vi "XML_Data.vi"(8 "Data Input Array":dbl[](array[numeric]), 9 "Data Tag Names Array":string[](array[string])=["DATA_1", "DATA_2", "DATA_3", "DATA_4"], 10 "XML File Path":path, 11 "DOM document in":refnum<k20>) -> (2 "XML Output":string, 3 "DOM document out":refnum<k20>)   [LabVIEW 2009]
doc: "Parses and Inserts a 1-D array of data into an XML file specified by the file path. The input XML file must have a DATA_SET node. Also, takes a 1-D array of strings to determine the node names for the data tags. The XML_Data VI can take 1-D arrays with 1-6 elements for both the numaric and string arrays, but can be modified to add up to 9 total. \n\nNOTE: If the string and numaric arrays are of different lengths the length of the numaric array will be used to determine the number of data nodes the XML file will have and data node names will be filled in with default values if needed."
uses:
  Program Files/National Instruments/LabVIEW 2009/resource/objmgr/DOMUserDefRef.rc
  <vilib>/xml/NI_XML.lvlib
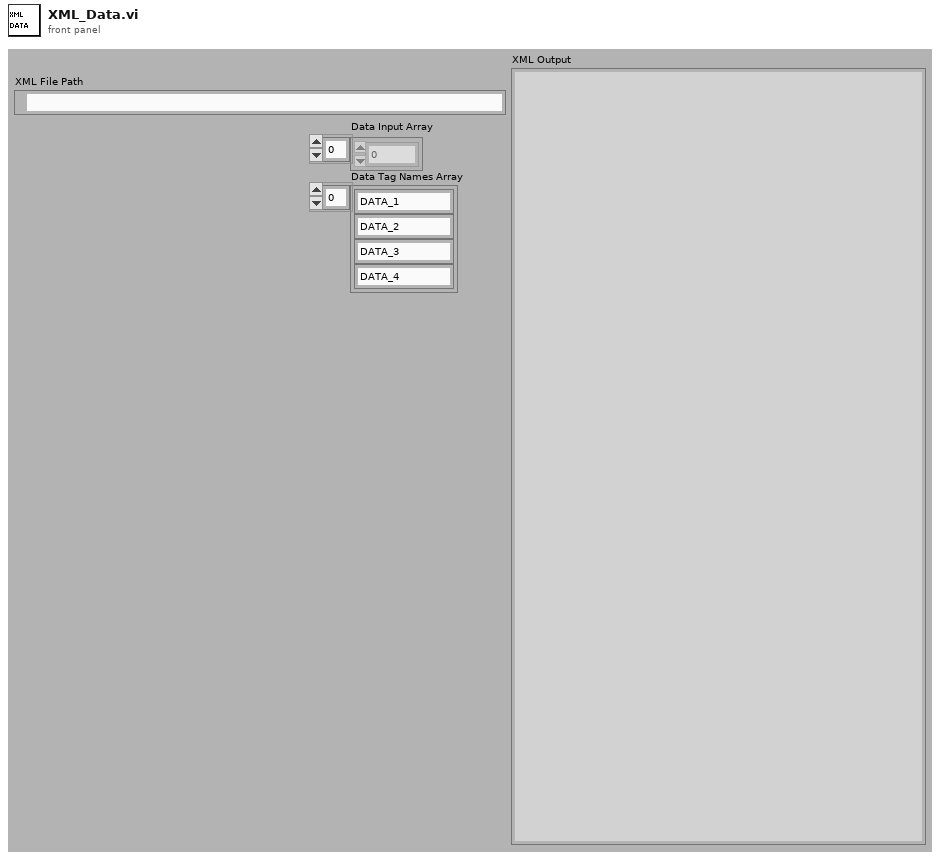
[diagram p1: front panel]
types:
  T1 = cluster{"Data Tag Names Array[0]":string, "Data Tag Names Array[1]":string, "Data Tag Names Array[2]":string, "Data Tag Names Array[3]":string, "Data Tag Names Array[4]":string, "Data Tag Names Array[5]":string, "Data Tag Names Array[6]":string, "Data Tag Names Array[7]":string, "Data Tag Names Array[8]":string}
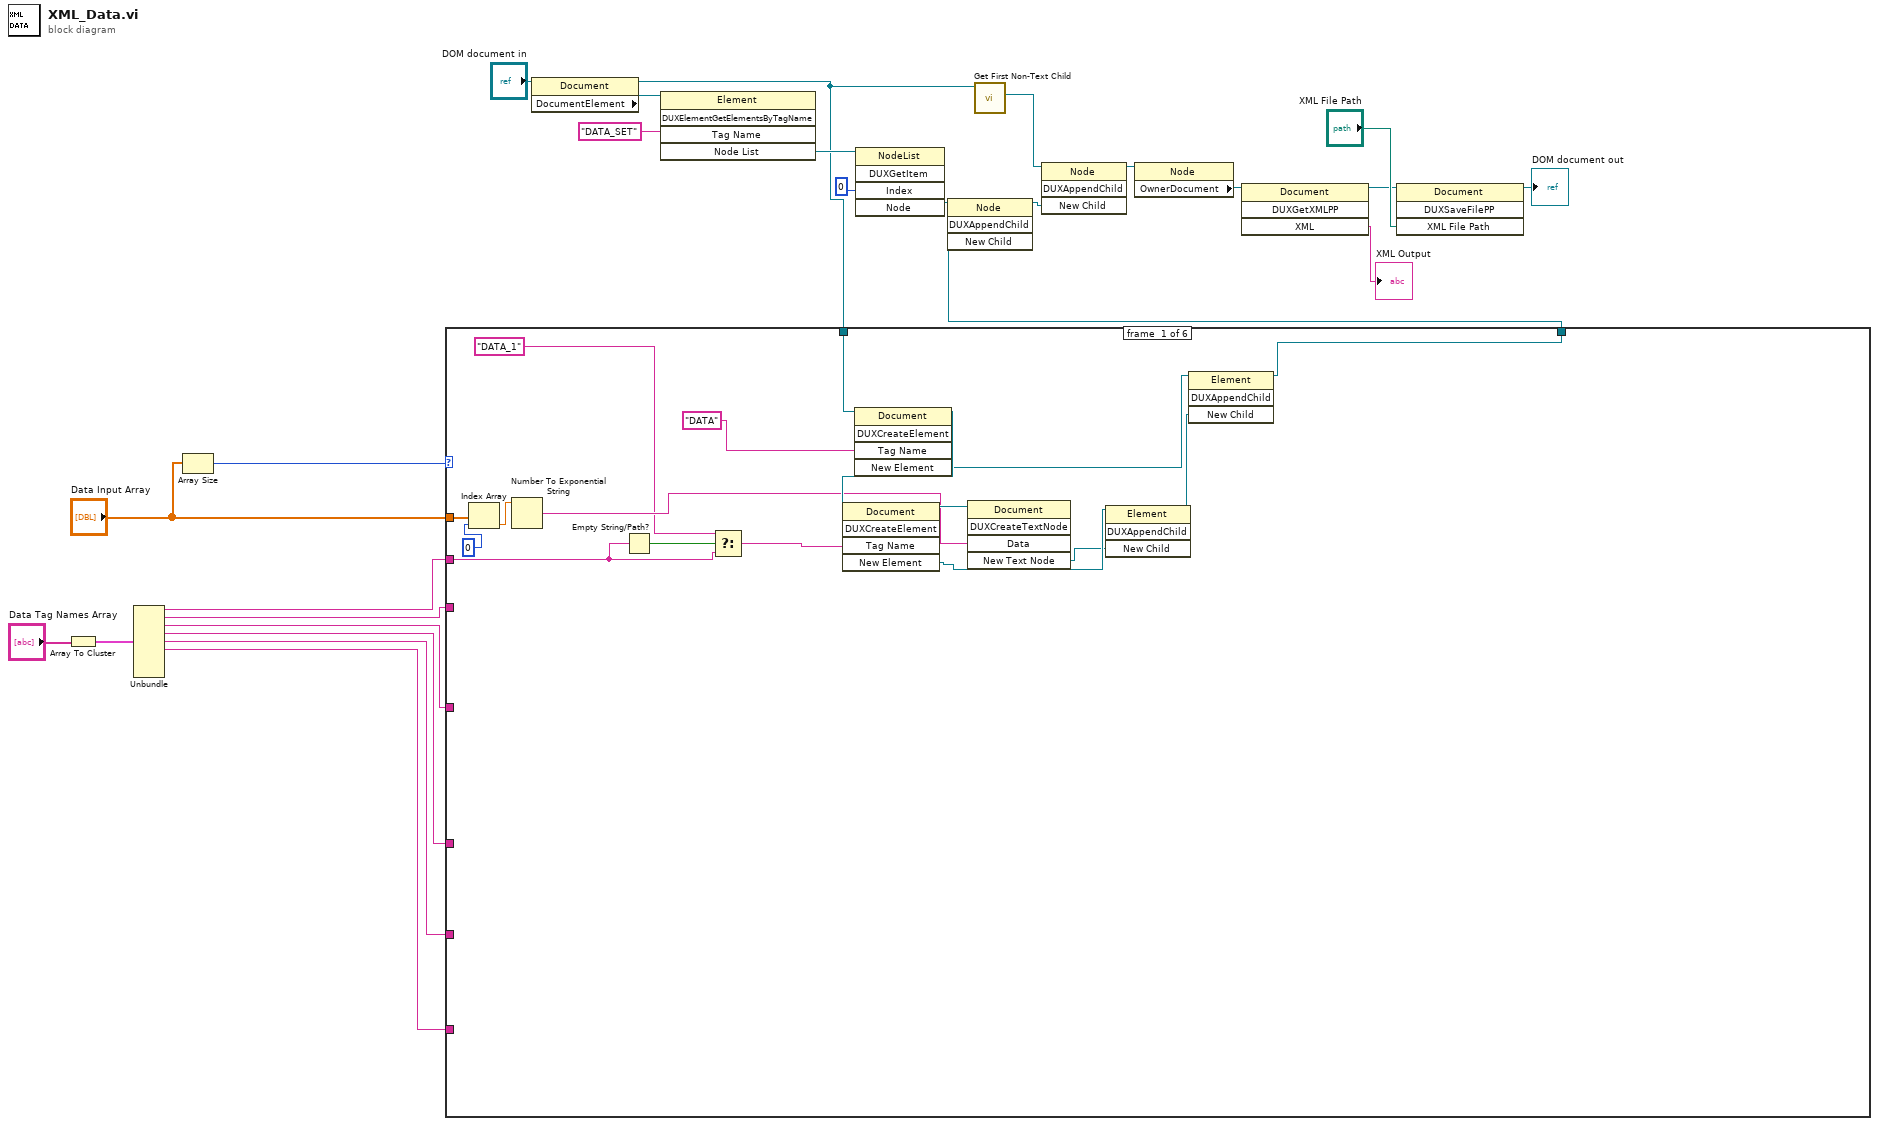
[diagram p0: block diagram]
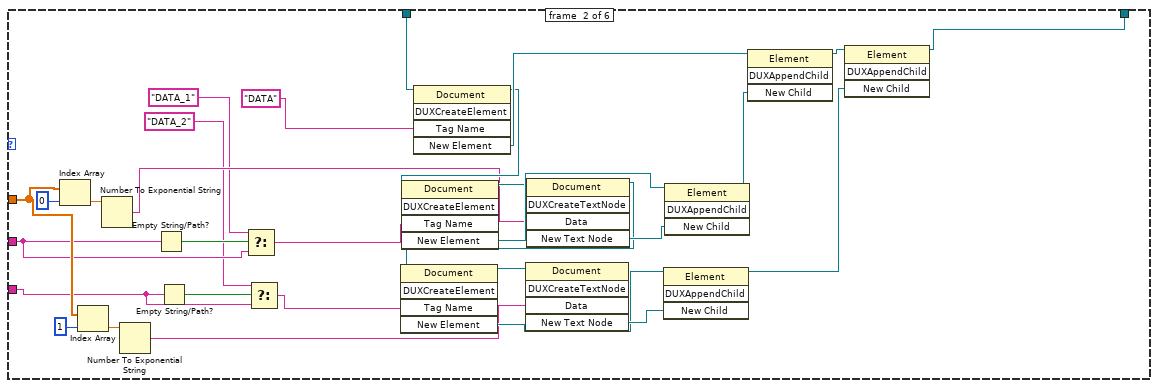
[diagram p2: hidden frame]
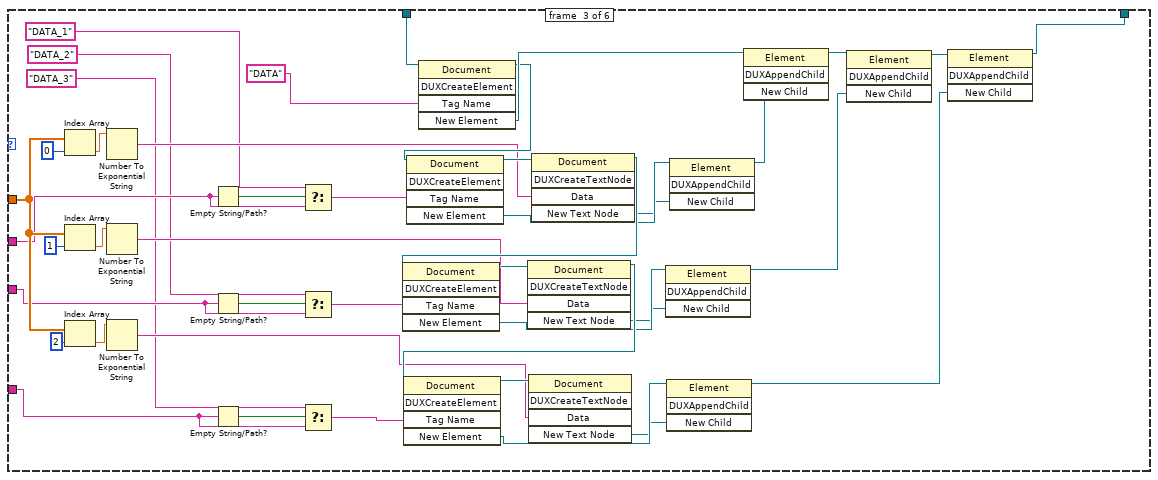
[diagram p3: hidden frame]
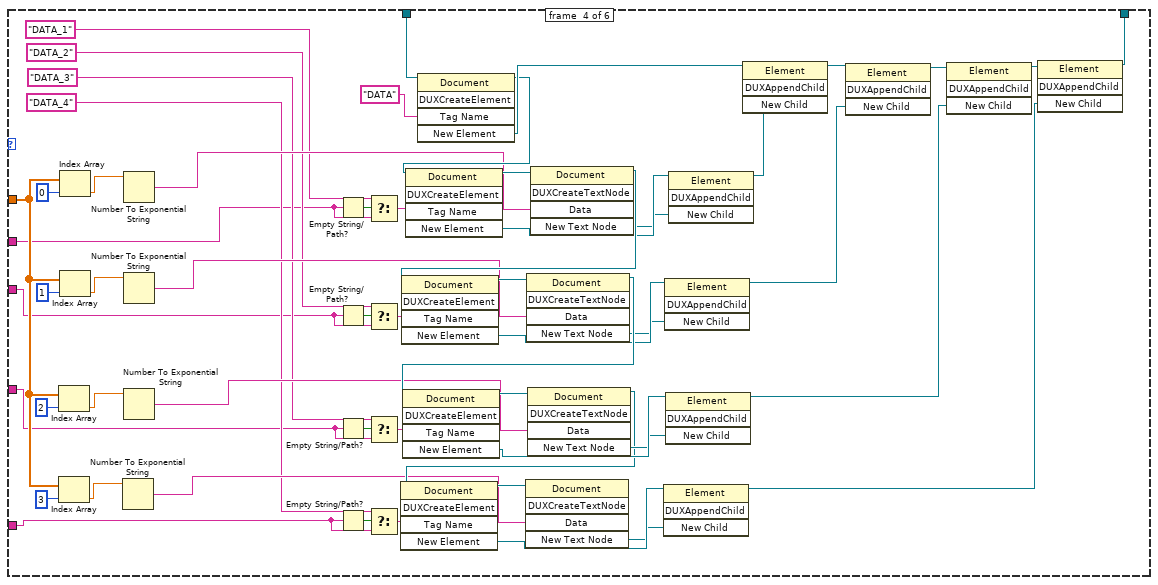
[diagram p4: hidden frame]
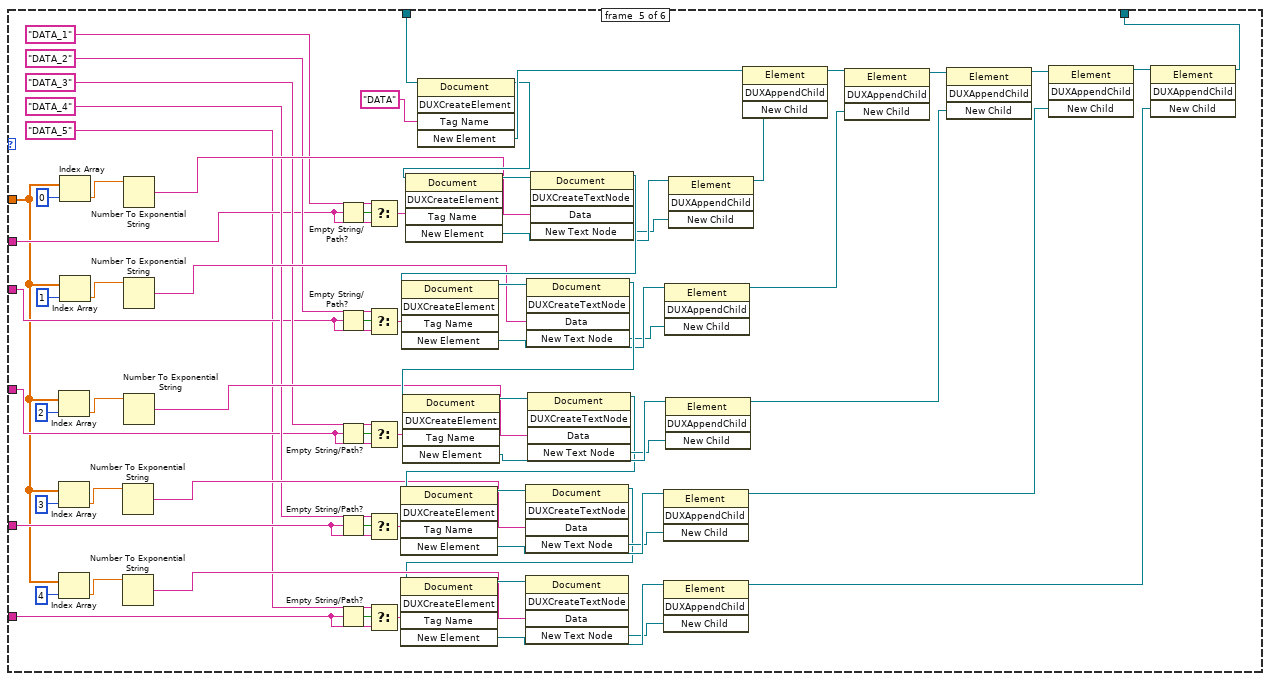
[diagram p5: hidden frame]
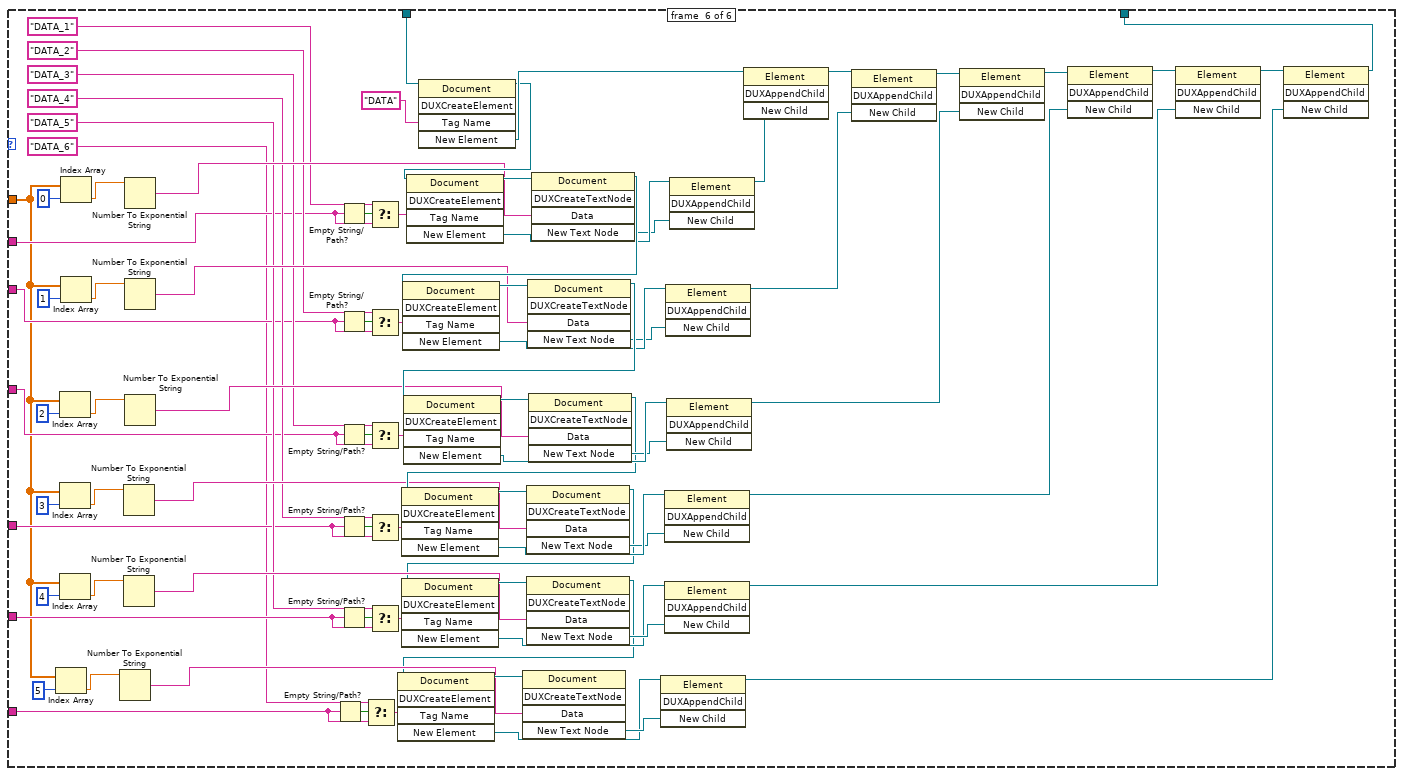
[diagram p6: hidden frame]
diagram:
  n1 = Array To Cluster(array="Data Tag Names Array") -> (cluster=w5:T1)
  n2 = Unbundle(w5) -> ("Data Tag Names Array[0]"=w10:string, "Data Tag Names Array[1]"=w9:string, "Data Tag Names Array[2]"=w8:string, "Data Tag Names Array[3]"=w7:string, "Data Tag Names Array[4]"=w4:string, "Data Tag Names Array[5]"=w3:string)  [unwired: 3 out]
  n3 = Array Size(array="Data Input Array") -> (size(s)=w18:i32)
  n4 = property class="Document"(reference="DOM document in") -> (reference out=w12:refnum<k20>, "DocumentElement"=w14:refnum<k20>)  [unwired: 1 in, 1 out]
  n5 = case shown="6" w18 {
    tunnel: w12 -> [w43 w60 w116 w153 w193 w263]
    tunnel: [w37 w59 w115 w146 w174 w242] -> w20
    tunnel: "Data Input Array" -> [w33 w55 w86 w137 w179 w248]
    tunnel: w10 -> [w29 w50 w82 w120 w192 w262]
    tunnel: w9 -> [_ w46 w78 w119 w191 w261]
    tunnel: w8 -> [_ _ w74 w118 w190 w260]
    tunnel: w7 -> [_ _ _ w117 w189 w259]
    tunnel: w4 -> [_ _ _ _ w178 w258]
    tunnel: w3 -> [_ _ _ _ _ w247]
    frame #0 {
      n6 = Index Array(array=w33, index=0) -> (element=w32:dbl)
      n7 = Number To Exponential String(number=w32) -> (E-format string=w31:string)  [unwired: 3 in]
      n8 = Empty String/Path?(string/path=w29) -> (empty?=w30:bool)
      n9 = Select(t="DATA_1", s=w30, f=w29) -> (s? t:f=w27:string)
      n10 = invoke class="Document" method="DUXCreateElement"(reference=w43, "Tag Name"="DATA") -> (reference out=w42:refnum<k20>, "New Element"=w36:refnum<k20>)  [unwired: 3 in, 3 out]
      n11 = invoke class="Document" method="DUXCreateElement"(reference=w42, "Tag Name"=w27) -> (reference out=w41:refnum<k20>, "New Element"=w40:refnum<k20>)  [unwired: 3 in, 3 out]
      n12 = invoke class="Document" method="DUXCreateTextNode"(reference=w41, "Data"=w31) -> ("New Text Node"=w39:refnum<k20>)  [unwired: 3 in, 4 out]
      n13 = invoke class="Element" method="DUXAppendChild"(reference=w40, "New Child"=w39) -> (reference out=w38:refnum<k20>)  [unwired: 2 in, 3 out]
      n14 = invoke class="Element" method="DUXAppendChild"(reference=w36, "New Child"=w38) -> (reference out=w37:refnum<k20>)  [unwired: 2 in, 3 out]
    }
    frame #1 {
      n15 = Index Array(array=w55, index=0) -> (element=w57:dbl)
      n16 = Index Array(array=w55, index=1) -> (element=w54:dbl)
      n17 = Number To Exponential String(number=w57) -> (E-format string=w53:string)  [unwired: 3 in]
      n18 = Number To Exponential String(number=w54) -> (E-format string=w52:string)  [unwired: 3 in]
      n19 = Empty String/Path?(string/path=w50) -> (empty?=w51:bool)
      n20 = Empty String/Path?(string/path=w46) -> (empty?=w47:bool)
      n21 = Select(t="DATA_1", s=w51, f=w50) -> (s? t:f=w48:string)
      n22 = Select(t="DATA_2", s=w47, f=w46) -> (s? t:f=w44:string)
      n23 = invoke class="Document" method="DUXCreateElement"(reference=w60, "Tag Name"="DATA") -> (reference out=w62:refnum<k20>, "New Element"=w70:refnum<k20>)  [unwired: 3 in, 3 out]
      n24 = invoke class="Document" method="DUXCreateElement"(reference=w62, "Tag Name"=w48) -> (reference out=w63:refnum<k20>, "New Element"=w66:refnum<k20>)  [unwired: 3 in, 3 out]
      n25 = invoke class="Document" method="DUXCreateTextNode"(reference=w63, "Data"=w53) -> (reference out=w64:refnum<k20>, "New Text Node"=w67:refnum<k20>)  [unwired: 3 in, 3 out]
      n26 = invoke class="Document" method="DUXCreateElement"(reference=w64, "Tag Name"=w44) -> (reference out=w65:refnum<k20>, "New Element"=w68:refnum<k20>)  [unwired: 3 in, 3 out]
      n27 = invoke class="Document" method="DUXCreateTextNode"(reference=w65, "Data"=w52) -> ("New Text Node"=w69:refnum<k20>)  [unwired: 3 in, 4 out]
      n28 = invoke class="Element" method="DUXAppendChild"(reference=w68, "New Child"=w69) -> (reference out=w72:refnum<k20>)  [unwired: 2 in, 3 out]
      n29 = invoke class="Element" method="DUXAppendChild"(reference=w66, "New Child"=w67) -> (reference out=w71:refnum<k20>)  [unwired: 2 in, 3 out]
      n30 = invoke class="Element" method="DUXAppendChild"(reference=w70, "New Child"=w71) -> (reference out=w73:refnum<k20>)  [unwired: 2 in, 3 out]
      n31 = invoke class="Element" method="DUXAppendChild"(reference=w73, "New Child"=w72) -> (reference out=w59:refnum<k20>)  [unwired: 2 in, 3 out]
    }
    frame #2 {
      n32 = Index Array(array=w86, index=0) -> (element=w93:dbl)
      n33 = Index Array(array=w86, index=1) -> (element=w92:dbl)
      n34 = Index Array(array=w86, index=2) -> (element=w88:dbl)
      n35 = Number To Exponential String(number=w93) -> (E-format string=w90:string)  [unwired: 3 in]
      n36 = Number To Exponential String(number=w92) -> (E-format string=w91:string)  [unwired: 3 in]
      n37 = Number To Exponential String(number=w88) -> (E-format string=w87:string)  [unwired: 3 in]
      n38 = Empty String/Path?(string/path=w82) -> (empty?=w84:bool)
      n39 = Empty String/Path?(string/path=w78) -> (empty?=w79:bool)
      n40 = Empty String/Path?(string/path=w74) -> (empty?=w75:bool)
      n41 = Select(t="DATA_1", s=w84, f=w82) -> (s? t:f=w85:string)
      n42 = Select(t="DATA_2", s=w79, f=w78) -> (s? t:f=w81:string)
      n43 = Select(t="DATA_3", s=w75, f=w74) -> (s? t:f=w77:string)
      n44 = invoke class="Document" method="DUXCreateElement"(reference=w116, "Tag Name"="DATA") -> (reference out=w108:refnum<k20>, "New Element"=w109:refnum<k20>)  [unwired: 3 in, 3 out]
      n45 = invoke class="Document" method="DUXCreateElement"(reference=w108, "Tag Name"=w85) -> (reference out=w107:refnum<k20>, "New Element"=w100:refnum<k20>)  [unwired: 3 in, 3 out]
      n46 = invoke class="Document" method="DUXCreateTextNode"(reference=w107, "Data"=w90) -> (reference out=w106:refnum<k20>, "New Text Node"=w99:refnum<k20>)  [unwired: 3 in, 3 out]
      n47 = invoke class="Document" method="DUXCreateElement"(reference=w106, "Tag Name"=w81) -> (reference out=w105:refnum<k20>, "New Element"=w101:refnum<k20>)  [unwired: 3 in, 3 out]
      n48 = invoke class="Document" method="DUXCreateTextNode"(reference=w105, "Data"=w91) -> (reference out=w104:refnum<k20>, "New Text Node"=w98:refnum<k20>)  [unwired: 3 in, 3 out]
      n49 = invoke class="Document" method="DUXCreateElement"(reference=w104, "Tag Name"=w77) -> (reference out=w103:refnum<k20>, "New Element"=w102:refnum<k20>)  [unwired: 3 in, 3 out]
      n50 = invoke class="Document" method="DUXCreateTextNode"(reference=w103, "Data"=w87) -> ("New Text Node"=w97:refnum<k20>)  [unwired: 3 in, 4 out]
      n51 = invoke class="Element" method="DUXAppendChild"(reference=w101, "New Child"=w98) -> (reference out=w111:refnum<k20>)  [unwired: 2 in, 3 out]
      n52 = invoke class="Element" method="DUXAppendChild"(reference=w102, "New Child"=w97) -> (reference out=w112:refnum<k20>)  [unwired: 2 in, 3 out]
      n53 = invoke class="Element" method="DUXAppendChild"(reference=w100, "New Child"=w99) -> (reference out=w110:refnum<k20>)  [unwired: 2 in, 3 out]
      n54 = invoke class="Element" method="DUXAppendChild"(reference=w109, "New Child"=w110) -> (reference out=w113:refnum<k20>)  [unwired: 2 in, 3 out]
      n55 = invoke class="Element" method="DUXAppendChild"(reference=w113, "New Child"=w111) -> (reference out=w114:refnum<k20>)  [unwired: 2 in, 3 out]
      n56 = invoke class="Element" method="DUXAppendChild"(reference=w114, "New Child"=w112) -> (reference out=w115:refnum<k20>)  [unwired: 2 in, 3 out]
    }
    frame #3 {
      n57 = Index Array(array=w137, index=2) -> (element=w140:dbl)
      n58 = Index Array(array=w137, index=3) -> (element=w138:dbl)
      n59 = Index Array(array=w137, index=0) -> (element=w144:dbl)
      n60 = Index Array(array=w137, index=1) -> (element=w142:dbl)
      n61 = Number To Exponential String(number=w138) -> (E-format string=w136:string)  [unwired: 3 in]
      n62 = Number To Exponential String(number=w144) -> (E-format string=w133:string)  [unwired: 3 in]
      n63 = Number To Exponential String(number=w142) -> (E-format string=w134:string)  [unwired: 3 in]
      n64 = Number To Exponential String(number=w140) -> (E-format string=w135:string)  [unwired: 3 in]
      n65 = Empty String/Path?(string/path=w120) -> (empty?=w131:bool)
      n66 = Empty String/Path?(string/path=w119) -> (empty?=w126:bool)
      n67 = Empty String/Path?(string/path=w118) -> (empty?=w125:bool)
      n68 = Empty String/Path?(string/path=w117) -> (empty?=w124:bool)
      n69 = Select(t="DATA_1", s=w131, f=w120) -> (s? t:f=w132:string)
      n70 = Select(t="DATA_2", s=w126, f=w119) -> (s? t:f=w127:string)
      n71 = Select(t="DATA_3", s=w125, f=w118) -> (s? t:f=w128:string)
      n72 = Select(t="DATA_4", s=w124, f=w117) -> (s? t:f=w129:string)
      n73 = invoke class="Document" method="DUXCreateElement"(reference=w153, "Tag Name"="DATA") -> (reference out=w166:refnum<k20>, "New Element"=w167:refnum<k20>)  [unwired: 3 in, 3 out]
      n74 = invoke class="Document" method="DUXCreateElement"(reference=w166, "Tag Name"=w132) -> (reference out=w165:refnum<k20>, "New Element"=w158:refnum<k20>)  [unwired: 3 in, 3 out]
      n75 = invoke class="Document" method="DUXCreateTextNode"(reference=w165, "Data"=w133) -> (reference out=w164:refnum<k20>, "New Text Node"=w157:refnum<k20>)  [unwired: 3 in, 3 out]
      n76 = invoke class="Document" method="DUXCreateElement"(reference=w164, "Tag Name"=w127) -> (reference out=w163:refnum<k20>, "New Element"=w159:refnum<k20>)  [unwired: 3 in, 3 out]
      n77 = invoke class="Document" method="DUXCreateTextNode"(reference=w163, "Data"=w134) -> (reference out=w162:refnum<k20>, "New Text Node"=w156:refnum<k20>)  [unwired: 3 in, 3 out]
      n78 = invoke class="Document" method="DUXCreateElement"(reference=w162, "Tag Name"=w128) -> (reference out=w161:refnum<k20>, "New Element"=w160:refnum<k20>)  [unwired: 3 in, 3 out]
      n79 = invoke class="Document" method="DUXCreateTextNode"(reference=w161, "Data"=w135) -> (reference out=w152:refnum<k20>, "New Text Node"=w155:refnum<k20>)  [unwired: 3 in, 3 out]
      n80 = invoke class="Document" method="DUXCreateElement"(reference=w152, "Tag Name"=w129) -> (reference out=w151:refnum<k20>, "New Element"=w150:refnum<k20>)  [unwired: 3 in, 3 out]
      n81 = invoke class="Document" method="DUXCreateTextNode"(reference=w151, "Data"=w136) -> ("New Text Node"=w149:refnum<k20>)  [unwired: 3 in, 4 out]
      n82 = invoke class="Element" method="DUXAppendChild"(reference=w150, "New Child"=w149) -> (reference out=w148:refnum<k20>)  [unwired: 2 in, 3 out]
      n83 = invoke class="Element" method="DUXAppendChild"(reference=w159, "New Child"=w156) -> (reference out=w169:refnum<k20>)  [unwired: 2 in, 3 out]
      n84 = invoke class="Element" method="DUXAppendChild"(reference=w160, "New Child"=w155) -> (reference out=w170:refnum<k20>)  [unwired: 2 in, 3 out]
      n85 = invoke class="Element" method="DUXAppendChild"(reference=w158, "New Child"=w157) -> (reference out=w168:refnum<k20>)  [unwired: 2 in, 3 out]
      n86 = invoke class="Element" method="DUXAppendChild"(reference=w167, "New Child"=w168) -> (reference out=w171:refnum<k20>)  [unwired: 2 in, 3 out]
      n87 = invoke class="Element" method="DUXAppendChild"(reference=w171, "New Child"=w169) -> (reference out=w172:refnum<k20>)  [unwired: 2 in, 3 out]
      n88 = invoke class="Element" method="DUXAppendChild"(reference=w172, "New Child"=w170) -> (reference out=w147:refnum<k20>)  [unwired: 2 in, 3 out]
      n89 = invoke class="Element" method="DUXAppendChild"(reference=w147, "New Child"=w148) -> (reference out=w146:refnum<k20>)  [unwired: 2 in, 3 out]
    }
    frame #4 {
      n90 = Index Array(array=w179, index=2) -> (element=w212:dbl)
      n91 = Index Array(array=w179, index=3) -> (element=w210:dbl)
      n92 = Index Array(array=w179, index=4) -> (element=w184:dbl)
      n93 = Index Array(array=w179, index=0) -> (element=w216:dbl)
      n94 = Index Array(array=w179, index=1) -> (element=w214:dbl)
      n95 = Number To Exponential String(number=w210) -> (E-format string=w209:string)  [unwired: 3 in]
      n96 = Number To Exponential String(number=w184) -> (E-format string=w183:string)  [unwired: 3 in]
      n97 = Number To Exponential String(number=w216) -> (E-format string=w206:string)  [unwired: 3 in]
      n98 = Number To Exponential String(number=w214) -> (E-format string=w207:string)  [unwired: 3 in]
      n99 = Number To Exponential String(number=w212) -> (E-format string=w208:string)  [unwired: 3 in]
      n100 = Empty String/Path?(string/path=w192) -> (empty?=w204:bool)
      n101 = Empty String/Path?(string/path=w191) -> (empty?=w199:bool)
      n102 = Empty String/Path?(string/path=w190) -> (empty?=w198:bool)
      n103 = Empty String/Path?(string/path=w189) -> (empty?=w197:bool)
      n104 = Empty String/Path?(string/path=w178) -> (empty?=w181:bool)
      n105 = Select(t="DATA_1", s=w204, f=w192) -> (s? t:f=w205:string)
      n106 = Select(t="DATA_2", s=w199, f=w191) -> (s? t:f=w200:string)
      n107 = Select(t="DATA_3", s=w198, f=w190) -> (s? t:f=w201:string)
      n108 = Select(t="DATA_4", s=w197, f=w189) -> (s? t:f=w202:string)
      n109 = Select(t="DATA_5", s=w181, f=w178) -> (s? t:f=w182:string)
      n110 = invoke class="Document" method="DUXCreateElement"(reference=w193, "Tag Name"="DATA") -> (reference out=w236:refnum<k20>, "New Element"=w237:refnum<k20>)  [unwired: 3 in, 3 out]
      n111 = invoke class="Document" method="DUXCreateElement"(reference=w236, "Tag Name"=w205) -> (reference out=w235:refnum<k20>, "New Element"=w228:refnum<k20>)  [unwired: 3 in, 3 out]
      n112 = invoke class="Document" method="DUXCreateTextNode"(reference=w235, "Data"=w206) -> (reference out=w234:refnum<k20>, "New Text Node"=w227:refnum<k20>)  [unwired: 3 in, 3 out]
      n113 = invoke class="Document" method="DUXCreateElement"(reference=w234, "Tag Name"=w200) -> (reference out=w233:refnum<k20>, "New Element"=w229:refnum<k20>)  [unwired: 3 in, 3 out]
      n114 = invoke class="Document" method="DUXCreateTextNode"(reference=w233, "Data"=w207) -> (reference out=w232:refnum<k20>, "New Text Node"=w226:refnum<k20>)  [unwired: 3 in, 3 out]
      n115 = invoke class="Document" method="DUXCreateElement"(reference=w232, "Tag Name"=w201) -> (reference out=w231:refnum<k20>, "New Element"=w230:refnum<k20>)  [unwired: 3 in, 3 out]
      n116 = invoke class="Document" method="DUXCreateTextNode"(reference=w231, "Data"=w208) -> (reference out=w223:refnum<k20>, "New Text Node"=w225:refnum<k20>)  [unwired: 3 in, 3 out]
      n117 = invoke class="Document" method="DUXCreateElement"(reference=w223, "Tag Name"=w202) -> (reference out=w222:refnum<k20>, "New Element"=w221:refnum<k20>)  [unwired: 3 in, 3 out]
      n118 = invoke class="Document" method="DUXCreateTextNode"(reference=w222, "Data"=w209) -> (reference out=w180:refnum<k20>, "New Text Node"=w220:refnum<k20>)  [unwired: 3 in, 3 out]
      n119 = invoke class="Document" method="DUXCreateElement"(reference=w180, "Tag Name"=w182) -> (reference out=w188:refnum<k20>, "New Element"=w187:refnum<k20>)  [unwired: 3 in, 3 out]
      n120 = invoke class="Document" method="DUXCreateTextNode"(reference=w188, "Data"=w183) -> ("New Text Node"=w186:refnum<k20>)  [unwired: 3 in, 4 out]
      n121 = invoke class="Element" method="DUXAppendChild"(reference=w221, "New Child"=w220) -> (reference out=w219:refnum<k20>)  [unwired: 2 in, 3 out]
      n122 = invoke class="Element" method="DUXAppendChild"(reference=w187, "New Child"=w186) -> (reference out=w176:refnum<k20>)  [unwired: 2 in, 3 out]
      n123 = invoke class="Element" method="DUXAppendChild"(reference=w229, "New Child"=w226) -> (reference out=w238:refnum<k20>)  [unwired: 2 in, 3 out]
      n124 = invoke class="Element" method="DUXAppendChild"(reference=w230, "New Child"=w225) -> (reference out=w239:refnum<k20>)  [unwired: 2 in, 3 out]
      n125 = invoke class="Element" method="DUXAppendChild"(reference=w228, "New Child"=w227) -> (reference out=w173:refnum<k20>)  [unwired: 2 in, 3 out]
      n126 = invoke class="Element" method="DUXAppendChild"(reference=w237, "New Child"=w173) -> (reference out=w240:refnum<k20>)  [unwired: 2 in, 3 out]
      n127 = invoke class="Element" method="DUXAppendChild"(reference=w240, "New Child"=w238) -> (reference out=w241:refnum<k20>)  [unwired: 2 in, 3 out]
      n128 = invoke class="Element" method="DUXAppendChild"(reference=w241, "New Child"=w239) -> (reference out=w218:refnum<k20>)  [unwired: 2 in, 3 out]
      n129 = invoke class="Element" method="DUXAppendChild"(reference=w218, "New Child"=w219) -> (reference out=w175:refnum<k20>)  [unwired: 2 in, 3 out]
      n130 = invoke class="Element" method="DUXAppendChild"(reference=w175, "New Child"=w176) -> (reference out=w174:refnum<k20>)  [unwired: 2 in, 3 out]
    }
    frame #5 {
      n131 = Index Array(array=w248, index=5) -> (element=w253:dbl)
      n132 = Index Array(array=w248, index=2) -> (element=w294:dbl)
      n133 = Index Array(array=w248, index=3) -> (element=w292:dbl)
      n134 = Index Array(array=w248, index=4) -> (element=w272:dbl)
      n135 = Index Array(array=w248, index=0) -> (element=w298:dbl)
      n136 = Index Array(array=w248, index=1) -> (element=w296:dbl)
      n137 = Number To Exponential String(number=w253) -> (E-format string=w252:string)  [unwired: 3 in]
      n138 = Number To Exponential String(number=w292) -> (E-format string=w291:string)  [unwired: 3 in]
      n139 = Number To Exponential String(number=w272) -> (E-format string=w271:string)  [unwired: 3 in]
      n140 = Number To Exponential String(number=w298) -> (E-format string=w288:string)  [unwired: 3 in]
      n141 = Number To Exponential String(number=w296) -> (E-format string=w289:string)  [unwired: 3 in]
      n142 = Number To Exponential String(number=w294) -> (E-format string=w290:string)  [unwired: 3 in]
      n143 = Empty String/Path?(string/path=w247) -> (empty?=w250:bool)
      n144 = Empty String/Path?(string/path=w262) -> (empty?=w286:bool)
      n145 = Empty String/Path?(string/path=w261) -> (empty?=w281:bool)
      n146 = Empty String/Path?(string/path=w260) -> (empty?=w280:bool)
      n147 = Empty String/Path?(string/path=w259) -> (empty?=w279:bool)
      n148 = Empty String/Path?(string/path=w258) -> (empty?=w269:bool)
      n149 = Select(t="DATA_6", s=w250, f=w247) -> (s? t:f=w251:string)
      n150 = Select(t="DATA_1", s=w286, f=w262) -> (s? t:f=w287:string)
      n151 = Select(t="DATA_2", s=w281, f=w261) -> (s? t:f=w282:string)
      n152 = Select(t="DATA_3", s=w280, f=w260) -> (s? t:f=w283:string)
      n153 = Select(t="DATA_4", s=w279, f=w259) -> (s? t:f=w284:string)
      n154 = Select(t="DATA_5", s=w269, f=w258) -> (s? t:f=w270:string)
      n155 = invoke class="Document" method="DUXCreateElement"(reference=w263, "Tag Name"="DATA") -> (reference out=w318:refnum<k20>, "New Element"=w319:refnum<k20>)  [unwired: 3 in, 3 out]
      n156 = invoke class="Document" method="DUXCreateElement"(reference=w318, "Tag Name"=w287) -> (reference out=w317:refnum<k20>, "New Element"=w310:refnum<k20>)  [unwired: 3 in, 3 out]
      n157 = invoke class="Document" method="DUXCreateTextNode"(reference=w317, "Data"=w288) -> (reference out=w316:refnum<k20>, "New Text Node"=w309:refnum<k20>)  [unwired: 3 in, 3 out]
      n158 = invoke class="Document" method="DUXCreateElement"(reference=w316, "Tag Name"=w282) -> (reference out=w315:refnum<k20>, "New Element"=w311:refnum<k20>)  [unwired: 3 in, 3 out]
      n159 = invoke class="Document" method="DUXCreateTextNode"(reference=w315, "Data"=w289) -> (reference out=w314:refnum<k20>, "New Text Node"=w308:refnum<k20>)  [unwired: 3 in, 3 out]
      n160 = invoke class="Document" method="DUXCreateElement"(reference=w314, "Tag Name"=w283) -> (reference out=w313:refnum<k20>, "New Element"=w312:refnum<k20>)  [unwired: 3 in, 3 out]
      n161 = invoke class="Document" method="DUXCreateTextNode"(reference=w313, "Data"=w290) -> (reference out=w305:refnum<k20>, "New Text Node"=w307:refnum<k20>)  [unwired: 3 in, 3 out]
      n162 = invoke class="Document" method="DUXCreateElement"(reference=w305, "Tag Name"=w284) -> (reference out=w304:refnum<k20>, "New Element"=w303:refnum<k20>)  [unwired: 3 in, 3 out]
      n163 = invoke class="Document" method="DUXCreateTextNode"(reference=w304, "Data"=w291) -> (reference out=w268:refnum<k20>, "New Text Node"=w302:refnum<k20>)  [unwired: 3 in, 3 out]
      n164 = invoke class="Document" method="DUXCreateElement"(reference=w268, "Tag Name"=w270) -> (reference out=w275:refnum<k20>, "New Element"=w257:refnum<k20>)  [unwired: 3 in, 3 out]
      n165 = invoke class="Document" method="DUXCreateTextNode"(reference=w275, "Data"=w271) -> (reference out=w245:refnum<k20>, "New Text Node"=w274:refnum<k20>)  [unwired: 3 in, 3 out]
      n166 = invoke class="Document" method="DUXCreateElement"(reference=w245, "Tag Name"=w251) -> (reference out=w256:refnum<k20>, "New Element"=w249:refnum<k20>)  [unwired: 3 in, 3 out]
      n167 = invoke class="Document" method="DUXCreateTextNode"(reference=w256, "Data"=w252) -> ("New Text Node"=w255:refnum<k20>)  [unwired: 3 in, 4 out]
      n168 = invoke class="Element" method="DUXAppendChild"(reference=w249, "New Child"=w255) -> (reference out=w244:refnum<k20>)  [unwired: 2 in, 3 out]
      n169 = invoke class="Element" method="DUXAppendChild"(reference=w303, "New Child"=w302) -> (reference out=w301:refnum<k20>)  [unwired: 2 in, 3 out]
      n170 = invoke class="Element" method="DUXAppendChild"(reference=w257, "New Child"=w274) -> (reference out=w266:refnum<k20>)  [unwired: 2 in, 3 out]
      n171 = invoke class="Element" method="DUXAppendChild"(reference=w311, "New Child"=w308) -> (reference out=w320:refnum<k20>)  [unwired: 2 in, 3 out]
      n172 = invoke class="Element" method="DUXAppendChild"(reference=w312, "New Child"=w307) -> (reference out=w321:refnum<k20>)  [unwired: 2 in, 3 out]
      n173 = invoke class="Element" method="DUXAppendChild"(reference=w310, "New Child"=w309) -> (reference out=w264:refnum<k20>)  [unwired: 2 in, 3 out]
      n174 = invoke class="Element" method="DUXAppendChild"(reference=w319, "New Child"=w264) -> (reference out=w322:refnum<k20>)  [unwired: 2 in, 3 out]
      n175 = invoke class="Element" method="DUXAppendChild"(reference=w322, "New Child"=w320) -> (reference out=w323:refnum<k20>)  [unwired: 2 in, 3 out]
      n176 = invoke class="Element" method="DUXAppendChild"(reference=w323, "New Child"=w321) -> (reference out=w300:refnum<k20>)  [unwired: 2 in, 3 out]
      n177 = invoke class="Element" method="DUXAppendChild"(reference=w300, "New Child"=w301) -> (reference out=w265:refnum<k20>)  [unwired: 2 in, 3 out]
      n178 = invoke class="Element" method="DUXAppendChild"(reference=w265, "New Child"=w266) -> (reference out=w243:refnum<k20>)  [unwired: 2 in, 3 out]
      n179 = invoke class="Element" method="DUXAppendChild"(reference=w243, "New Child"=w244) -> (reference out=w242:refnum<k20>)  [unwired: 2 in, 3 out]
    }
  }
  n180 = invoke class="Element" method="DUXElementGetElementsByTagName"(reference=w14, "Tag Name"="DATA_SET") -> ("Node List"=w25:refnum<k20>)  [unwired: 3 in, 4 out]
  n181 = invoke class="NodeList" method="DUXGetItem"(reference=w25, "Index"=0) -> ("Node"=w23:refnum<k20>)  [unwired: 3 in, 4 out]
  n182 = invoke class="Node" method="DUXAppendChild"(reference=w23, "New Child"=w20) -> (reference out=w22:refnum<k20>)  [unwired: 2 in, 3 out]
  n183 = call <vilib>:"Get First Non-Text Child.vi"("node in"=w12) -> ("child node"=w21:refnum<k20>)  [unwired: 7 in, 3 out]
  n184 = invoke class="Node" method="DUXAppendChild"(reference=w21, "New Child"=w22) -> (reference out=w16:refnum<k20>)  [unwired: 2 in, 3 out]
  n185 = property class="Node"(reference=w16) -> ("OwnerDocument"=w15:refnum<k20>)  [unwired: 1 in, 2 out]
  n186 = invoke class="Document" method="DUXGetXMLPP"(reference=w15) -> (reference out=w1:refnum<k20>, "XML"=→"XML Output":string)  [unwired: 3 in, 2 out]
  n187 = invoke class="Document" method="DUXSaveFilePP"(reference=w1, "XML File Path"="XML File Path") -> (reference out=→"DOM document out":refnum<k20>)  [unwired: 2 in, 3 out]
